vi "Build Send.vi"(4 "BuildType":T2 items=["simple", "Dialog", "PVUpdate", "Dialog&PV", "Asynch", "AsynchDial", "Ack"], 6 "Wiring Spec":T1, 8 "error in (no error)":errorcluster, 10 "Send VI":refnum<vi>, 11 "CS++Actor in":refnum<class "CS++Actor.lvclass">) -> (0 "error out":errorcluster, 3 "CS++Actor out":refnum<class "CS++Actor.lvclass">)   [LabVIEW 2016, in "CS++Actor.lvlib" / "CS++Actor.lvclass"]
doc: "Creates the send.vi of the new message."
uses:
  CS++Actor.lvclass
  CSPP_MessageMakerMain/BuildType.ctl
  <vilib>/LabVIEW Icon API/lv_icon/Controls/Graphic.ctl
  CS++Actor.lvclass/CS++Actor.ctl
  <vilib>/Utility/traverseref.llb/TRef TravTarget.ctl
  <vilib>/Utility/miscctls.llb/LVPositionTypeDef.ctl
  <vilib>/LabVIEW Icon API/lv_icon/Classes/Icon/Icon.lvclass
  <vilib>/LabVIEW Icon API/lv_icon/Classes/Icon Framework/Icon Framework.lvclass
  <vilib>/Utility/traverseref.llb/VI Scripting - Traverse.lvlib
  <vilib>/LabVIEW Icon API/LabVIEW Icon API.lvlib
  CSPP_MessageMakerMain/CS++MessageMakerMain.lvclass
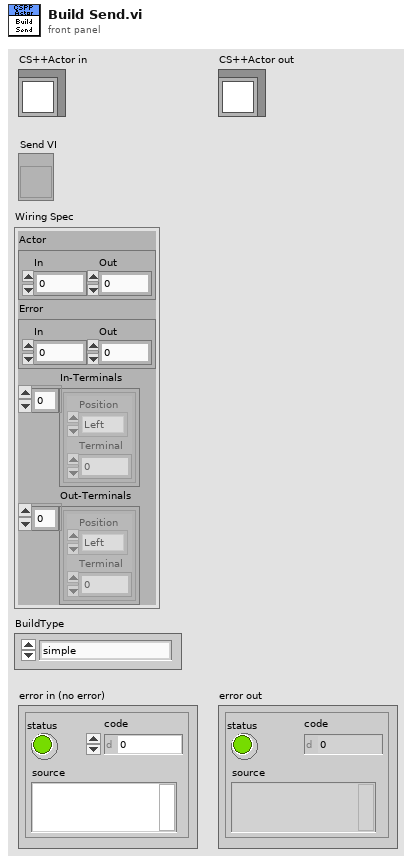
[diagram p1: front panel]
types:
  T1 = cluster{"Actor":cluster{"In":i32, "Out":i32}, "Error":cluster{"In":i32, "Out":i32}, "In-Terminals":cluster{"Position":enum16{"Left", "Top", "Bottom", "Right"}, "Terminal":i32}[], "Out-Terminals":cluster{"Position":enum16{"Left", "Top", "Bottom", "Right"}, "Terminal":i32}[]}
  T2 = typedef "CS++MessageMakerMain.lvlib/CS++MessageMakerMain.lvclass/BuildType.ctl" = u16
  T3 = typedef "Graphic.ctl" = cluster{"Rectangle":cluster{"left":i16, "top":i16, "right":i16, "bottom":i16}, "Path":path, "Image":picture, "Filter":string, "FileName":string}
  T4 = typedef "BodyText.ctl" = cluster{"Line 1 text":string, "Line 2 text":string, "Line 3 text":string, "Line 4 text":string, "Line 1 color":u32, "Line 2 color":u32, "Line 3 color":u32, "Line 4 color":u32, "Body Text Spec":cluster{"Font":T5, "Alignment":T6, "Size":u8}, "Center text vertically":bool, "Capitalize Text":bool}
  T5 = typedef "Font.ctl" = string
  T6 = typedef "Alignment.ctl" = u16
  T7 = typedef "TRef TravTarget.ctl" = enum16{"FP", "BD", "Other"}
  T8 = enum16{"Invalid Wire Rule", "Required", "Recommended", "Optional", "Dynamic Dispatch"}
  T9 = typedef "LVPositionTypeDef.ctl" = cluster{"Left":i32, "Top":i32}
  T10 = enum16{"Invalid Wire Rule", "Required", "Recommended", "Optional", "Dynamic Dispatch"}[]
  T11 = cluster{"Position":enum16{"Left", "Top", "Bottom", "Right"}, "Terminal":i32}[]
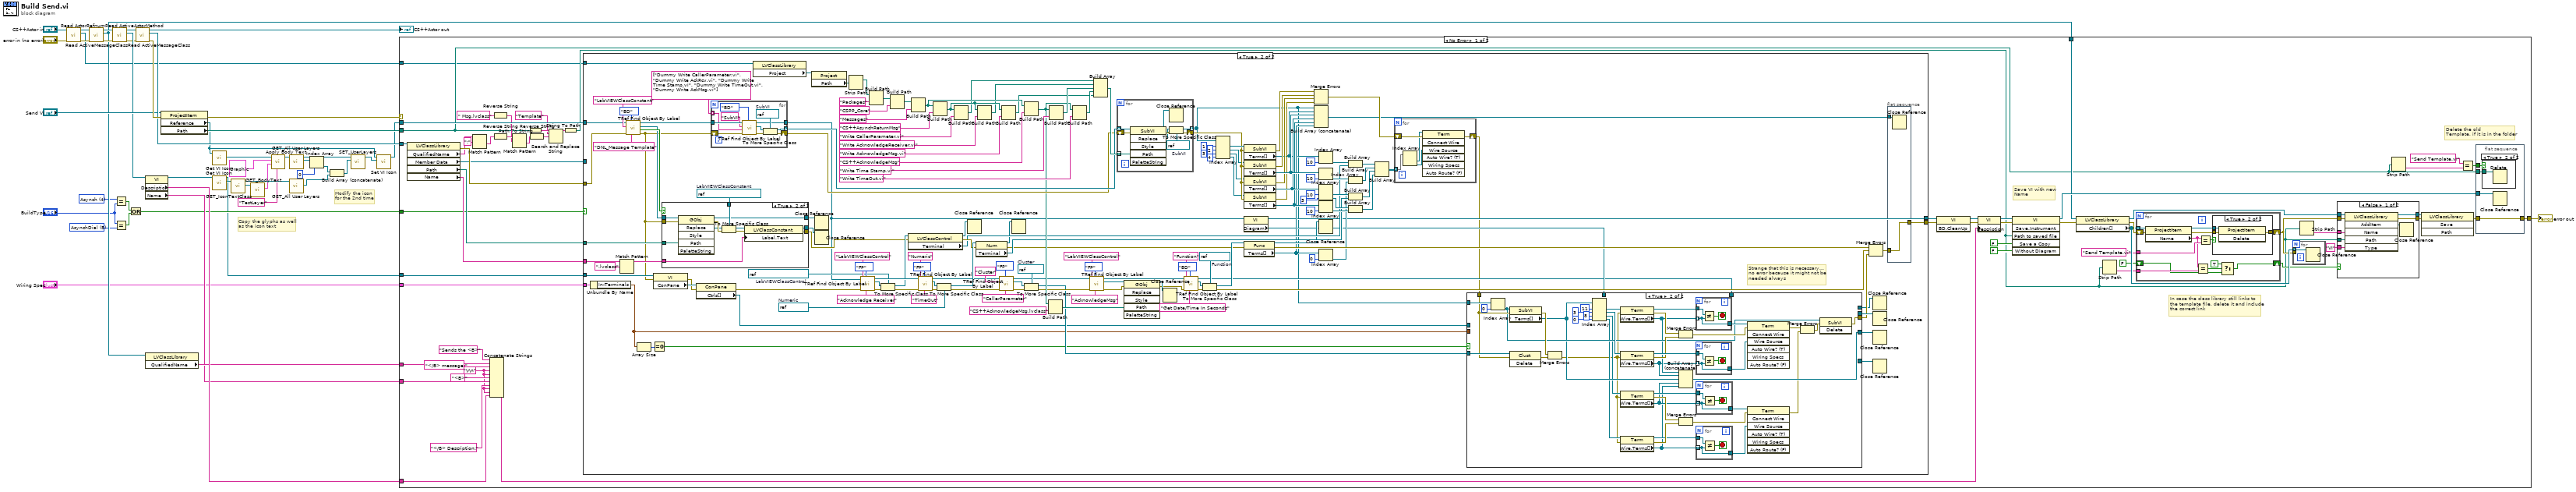
[diagram p0: block diagram]
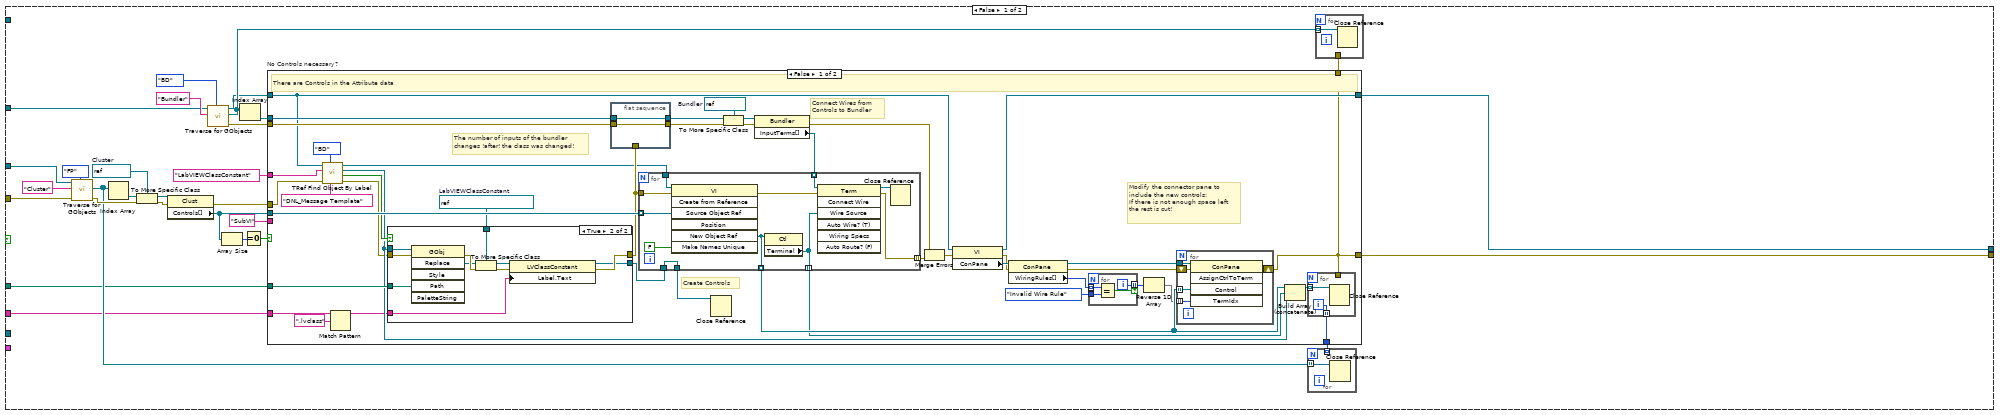
[diagram p3: hidden frame]
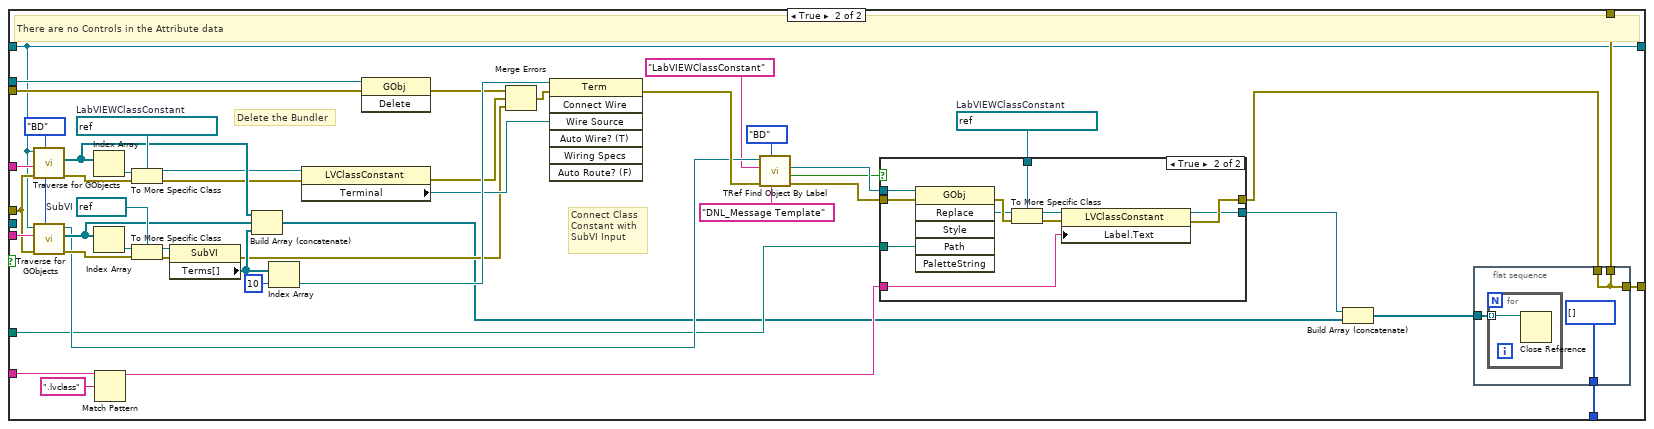
[diagram p5: hidden frame]
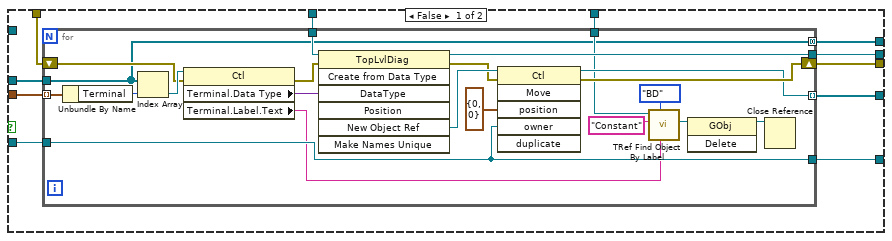
[diagram p8: hidden frame]
diagram:
  w2 = T2 5 items=["simple", "Dialog", "PVUpdate", "Dialog&PV", "Asynch", "AsynchDial", "Ack"] ("BuildType")
  w1 = T2 4 items=["simple", "Dialog", "PVUpdate", "Dialog&PV", "Asynch", "AsynchDial", "Ack"] ("BuildType")
  # "Copy the glyphs as well\nas the icon text"
  # "Modify the icon\nfor the 2nd time"
  n1 = call "Read ActorRefnum.vi"("error in (no error)"="error in (no error)", "CS++Actor in"="CS++Actor in") -> ("error out"=w6:errorcluster, "ActorRefnum"=w5:refnum<vi>, "CS++Actor out"=w8:refnum<class "CS++Actor.lvclass">)  [unwired: 7 in]
  n2 = call "Read ActiveMessageClass.vi"("error in (no error)"=w6, "CS++Actor in"=w8) -> ("error out"=w25:errorcluster, "ActiveMessageClass"=w22:refnum<vi>, "CS++Actor out"=w26:refnum<class "CS++Actor.lvclass">)  [unwired: 7 in]
  n3 = call "Read ActiveActorMethod.vi"("error in (no error)"=w25, "CS++Actor in"=w26) -> ("error out"=w27:errorcluster, "ActiveActorMethod"=w31:refnum<vi>, "CS++Actor out"=w28:refnum<class "CS++Actor.lvclass">)  [unwired: 7 in]
  n4 = Equal?(x=w1, y="BuildType") -> (x = y?=w12:bool)
  n5 = Equal?(x="BuildType", y=w2) -> (x = y?=w11:bool)
  n6 = Or(x=w12, y=w11) -> (x .or. y?=w10:bool)
  n7 = call "Read ActiveMessageClass.vi"("error in (no error)"=w27, "CS++Actor in"=w28) -> ("error out"=w43:errorcluster, "ActiveMessageClass"=w42:refnum<vi>, "CS++Actor out"=→"CS++Actor out":refnum<class "CS++Actor.lvclass">)  [unwired: 7 in]
  n8 = property class="VI"(reference=w31) -> (reference out=w30:refnum<vi>, "Description"=w29:string, "Name"=w23:string)  [unwired: 1 in, 1 out]
  n9 = property class="LVClassLibrary"(reference=w22) -> ("QualifiedName"=w24:string)  [unwired: 1 in, 2 out]
  n10 = property class="ProjectItem"(reference="Send VI", error in=w43) -> (error out=w46:errorcluster, "Reference"=w32:refnum<vi>, "Path"=w45:path)  [unwired: 1 out]
  n11 = call <vilib>:"Get VI Icon.vi"("VI Refnum in"=w32) -> ("Icon"=w18:refnum<class "Icon.lvclass">)  [unwired: 8 in, 2 out]
  n12 = call <vilib>:"Get VI Icon.vi"("VI Refnum in"=w30) -> ("Icon"=w20:refnum<class "Icon.lvclass">, "VI Refnum out"=w3:refnum<vi>)  [unwired: 8 in, 1 out]
  n13 = call-dynamic "GET_IconTextClass.vi"("Icon.lvclass in"=w20) -> ("Icon Framework.lvclass"=w21:refnum<class "Icon Framework.lvclass">, "Icon.lvclass out"=w19:refnum<class "Icon.lvclass">)  [unwired: 8 in, 1 out]
  n14 = call-dynamic "GET_BodyText.vi"("Icon Framework.lvclass in"=w21) -> ("Body Text"=w16:T4)  [unwired: 7 in, 3 out]
  n15 = call <vilib>:"Apply Body Text.vi"("Layer name"="TestLayer", "Body test"=w16, "Path & Icon"=T3 {"Rectangle"={"left"=0, "top"=0, "right"=0, "bottom"=0}, "Path"=path "", "Image"=bytes[0], "Filter"="", "FileName"=""}, "Icon in"=w18) -> ("Icon out"=w17:refnum<class "Icon.lvclass">)  [unwired: 5 in, 2 out]
  n16 = call-dynamic "GET_All User Layers.vi"("Icon.lvclass in"=w17) -> ("User Layer"=w39:refnum<class "Layer.lvclass">[], "Icon.lvclass out"=w40:refnum<class "Icon.lvclass">)  [unwired: 8 in, 1 out]
  n17 = call-dynamic "GET_All User Layers.vi"("Icon.lvclass in"=w19) -> ("User Layer"=w36:refnum<class "Layer.lvclass">[])  [unwired: 8 in, 2 out]
  n18 = Index Array(array=w39, index=0) -> (element=w37:refnum<class "Layer.lvclass">)
  n19 = Build Array (concatenate)(w37, w36) -> (w35:refnum<class "Layer.lvclass">[])
  n20 = call-dynamic "SET_UserLayers.vi"("Layers"=w35, "Icon.lvclass in"=w40) -> ("Icon.lvclass out"=w34:refnum<class "Icon.lvclass">)  [unwired: 8 in, 1 out]
  n21 = call <vilib>:"Set VI Icon.vi"("Icon"=w34, "VI Refnum in"=w32) -> ("VI Refnum out"=w33:refnum<vi>)  [unwired: 8 in, 1 out]
  n22 = case shown="No Error" w46 {
    selector: w46 -> [_ w596]
    tunnel: [w59 w596] -> w47
    tunnel: w42 -> [w60 _]
    tunnel: w33 -> [w106 _]
    tunnel: w45 -> [w57 _]
    tunnel: w29 -> [w80 _]
    tunnel: w24 -> [w72 _]
    tunnel: w23 -> [w83 _]
    tunnel: w22 -> [w75 _]
    tunnel: w10 -> [w51 _]
    tunnel: w5 -> [w50 _]
    tunnel: "Wiring Spec" -> [w49 _]
    tunnel: w3 -> [w48 _]
    frame No Error {
      w79 = "\r\n"
      # "In case the class library still links to\nthe template file, delete it and include\nthe correct link"
      # "Delete the old\nTemplate, if it is in the folder"
      # "Save VI with new\nName"
      n23 = property class="LVClassLibrary"(reference=w60) -> (error out=w107:errorcluster, "QualifiedName"=w100:string, "Member Data"=w101:refnum<vi>, "Path"=w62:path, "Name"=w52:string)  [unwired: 1 in, 1 out]
      n24 = Match Pattern(string=w100, regular expression=":") -> (after substring=w93:string)  [unwired: 1 in, 3 out]
      n25 = Concatenate Strings("Sends the <B>", w72, "</B> message.", w79, w79, "<B>" ("string"), w83, "</B> Description:" ("string"), w79, w79, w80) -> (w86:string)
      n26 = Reverse String(1:" Msg.lvclass" ("search string")) -> (0:w95:string)
      n27 = Reverse String(1:w93) -> (0:w97:string)
      n28 = Match Pattern(string=w97, regular expression=w95) -> (after substring=w96:string)  [unwired: 1 in, 3 out]
      n29 = Path To String(path=w57) -> (string=w104:string)
      n30 = Reverse String(1:w96) -> (0:w98:string)
      n31 = Search and Replace String(input string=w104, search string="Template", replace string=w98) -> (result string=w102:string)  [unwired: 5 in, 3 out]
      n32 = String To Path(string=w102) -> (path=w61:path)
      n33 = case shown="True" w51 {
        tunnel: w107 -> [w136 w438]
        tunnel: w106 -> [w125 w440]
        tunnel: w101 -> [w124 _]
        tunnel: [w123 w288] -> w91
        tunnel: w62 -> [w116 w432]
        tunnel: [w114 w304] -> w53
        tunnel: w52 -> [w113 w434]
        tunnel: w50 -> [_ w428]
        tunnel: w49 -> [_ w321]
        tunnel: w48 -> [_ w320]
        frame False {
          w138 = refnum<vi> refnum  # Cluster
          n34 = call <vilib>:"Traverse for GObjects.vi"("Traverse Target"=TRef_TravTarget."FP", "error in (no error)"=w136, "Class Name"="Cluster" ("name/order"), "VI Refnum"=w124) -> ("error out"=w137:errorcluster, "References"=w128:refnum<vi>[])  [unwired: 4 in, 2 out]
          n35 = Index Array(array=w128) -> (element=w139:refnum<vi>)  [unwired: 1 in]
          n36 = To More Specific Class(target class=w138, reference=w139, error in=w137) -> (specific class reference=w135:refnum<vi>, error out=w134:errorcluster)
          n37 = property class="Clust"(reference=w135, error in=w134) -> (error out=w133:errorcluster, "Controls[]"=w122:refnum<vi>[])  [unwired: 1 out]
          n38 = call <vilib>:"Traverse for GObjects.vi"("Traverse Target"=TRef_TravTarget."BD", "Class Name"="Bundler", "VI Refnum"=w125) -> ("error out"=w130:errorcluster, "References"=w127:refnum<vi>[], "dup VI Refnum"=w115:refnum<vi>)  [unwired: 5 in, 1 out]
          n39 = Array Size(array=w122) -> (size(s)=w121:i32)
          n40 = Index Array(array=w127) -> (element=w120:refnum<vi>)  [unwired: 1 in]
          n41 = Equal To 0?(x=w121) -> (x = 0?=w119:bool)
          n42 = case "No Controls necessary?" shown="False" w119 {
            tunnel: w133 -> [w159 w256]
            tunnel: w130 -> [w145 w266]
            tunnel: [w179 w263] -> w129
            tunnel: [w163 w264] -> w126
            tunnel: [w163 w265] -> w123
            tunnel: w122 -> [w164 _]
            tunnel: w120 -> [w147 w267]
            tunnel: "LabVIEWClassConstant" ("Class Name") -> [w155 w262]
            tunnel: "SubVI" ("Class Name") -> [_ w257]
            tunnel: w116 -> [w176 w225]
            tunnel: w115 -> [w142 w221]
            tunnel: [w169 w221] -> w114
            tunnel: w113 -> [w151 w227]
            frame False {
              w149 = refnum<vi> refnum  # LabVIEWClassConstant
              w184 = refnum<vi> refnum  # Bundler
              # "The number of inputs of the bundler\nchanges !after! the class was changed!"
              # "Modify the connector pane to\ninclude the new controls:\nIf there is not enough space left\nthe rest is cut!"
              # "Connect Wires from\nControls to Bundler"
              # "Create Controls"
              # "There are Controls in the Attribute data"
              n43 = call <vilib>:"TRef Find Object By Label.vi"("Label"="DNL_Message Template", "Traverse Target"=TRef_TravTarget."BD", "error in (no error)"=w159, "Class Name"=w155, "VI Ref"=w142) -> ("error out"=w153:errorcluster, "Found?"=w156:bool, "Found Obj Ref"=w154:refnum<vi>, "dup VI Ref"=w143:refnum<vi>)  [unwired: 3 in]
              n44 = Match Pattern(string=w151, regular expression=".lvclass") -> (before substring=w150:string)  [unwired: 1 in, 3 out]
              n45 = case shown="True" w156 {
                tunnel: [w187 w192] -> w144
                tunnel: w176 -> [_ w198]
                tunnel: [_ w190] -> w175
                tunnel: w154 -> [_ w196]
                tunnel: w153 -> [w187 w197]
                tunnel: w150 -> [_ w188]
                tunnel: w149 -> [_ w189]
                frame False {
                }
                frame True {
                  n46 = invoke class="GObj" method="Replace"(reference=w196, error in=w197, "Path"=w198) -> (error out=w195:errorcluster, "Replace"=w194:refnum<vi>)  [unwired: 3 in, 4 out]
                  n47 = To More Specific Class(target class=w189, reference=w194, error in=w195) -> (specific class reference=w191:refnum<vi>, error out=w193:errorcluster)
                  n48 = property class="LVClassConstant"(reference=w191, error in=w193, "Label.Text"=w188) -> (reference out=w190:refnum<vi>, error out=w192:errorcluster)
                }
              }
              n49 = flat-sequence {
                tunnel: [w186] -> w148
                tunnel: w147 -> [w186]
                tunnel: [w185] -> w146
                tunnel: w145 -> [w185]
                tunnel: w144 -> [_]
                frame #0 {
                }
              }
              n50 = To More Specific Class(target class=w184, reference=w148, error in=w146) -> (specific class reference=w183:refnum<vi>, error out=w182:errorcluster)
              n51 = property class="Bundler"(reference=w183, error in=w182) -> (error out=w178:errorcluster, "InputTerms[]"=w181:refnum<vi>[])  [unwired: 1 out]
              n52 = for {
                tunnel: w164 -> [w220] mode=indexing
                tunnel: w143 -> [w218]
                tunnel: w144 -> [w217]
                tunnel: w181 -> [w215] mode=indexing
                tunnel: [w214] -> w180 mode=indexing
                tunnel: [w213] -> w161 mode=indexing
                tunnel: w175 -> [w211]
                tunnel: [w211] -> w174
                tunnel: [w210] -> w162 mode=indexing
                n53 = invoke class="VI" method="Create from Reference"(reference=w218, error in=w217, "Source Object Ref"=w220, "Make Names Unique"=FALSE ("Make Names Unique (F)")) -> (error out=w216:errorcluster, "New Object Ref"=w210:refnum<vi>)  [unwired: 3 in, 5 out]
                n54 = property class="Ctl"(reference=w210) -> ("Terminal"=w213:refnum<vi>)  [unwired: 1 in, 2 out]
                n55 = invoke class="Term" method="Connect Wire"(reference=w215, error in=w216, "Wire Source"=w213) -> (reference out=w212:refnum<vi>, error out=w214:errorcluster)  [unwired: 4 in, 5 out]
                n56 = Close Reference(reference=w212) -> ()  [unwired: 1 in, 1 out]
              }
              n57 = Close Reference(reference=w174) -> ()  [unwired: 1 in, 1 out]
              n58 = Merge Errors(w178, w180) -> (w173:errorcluster)
              n59 = property class="VI"(reference=w142, error in=w173) -> (reference out=w169:refnum<vi>, error out=w170:errorcluster, "ConPane"=w172:refnum<vi>)
              n60 = property class="ConPane"(reference=w172, error in=w170) -> (reference out=w171:refnum<vi>, error out=w166:errorcluster, "WiringRules[]"=w168:T10)
              n61 = for {
                tunnel: w168 -> [w207] mode=indexing
                tunnel: T8."Invalid Wire Rule" ("Wire Rule") -> [w206]
                tunnel: [w205] -> w165 mode=indexing if=w204
                i -> [w205]
                n62 = Equal?(x=w207, y=w206) -> (x = y?=w204:bool)
              }
              n63 = Reverse 1D Array(array=w165) -> (reversed array=w160:i32[])
              n64 = for {
                tunnel: w171 -> [w203]
                shift-right: [w201] -> w163
                shift-left: w166 -> [w202]
                tunnel: w160 -> [w200] mode=indexing
                tunnel: w162 -> [w199] mode=indexing
                n65 = invoke class="ConPane" method="AssignCtrlToTerm"(reference=w203, error in=w202, "Control"=w199, "TermIdx"=w200) -> (error out=w201:errorcluster)  [unwired: 1 in, 4 out]
              }
              n66 = Build Array (concatenate)(w162, w161, w154) -> (w177:refnum<vi>[])
              n67 = for {
                tunnel: w177 -> [w209] mode=indexing
                tunnel: [w208] -> w179 mode=indexing
                tunnel: w163 -> [_]
                i -> [w208]
                n68 = Close Reference(reference=w209) -> ()  [unwired: 1 in, 1 out]
              }
            }
            frame True {
              w234 = refnum<vi> refnum  # LabVIEWClassConstant
              w253 = refnum<vi> refnum  # SubVI
              w260 = refnum<vi> refnum  # LabVIEWClassConstant
              w258 = TRef_TravTarget."BD" ("Traverse Target")
              # "Connect Class\nConstant with\nSubVI Input"
              # "Delete the Bundler"
              # "There are no Controls in the Attribute data"
              n69 = call <vilib>:"Traverse for GObjects.vi"("Traverse Target"=w258, "error in (no error)"=w256, "Class Name"=w262, "VI Refnum"=w221) -> ("error out"=w259:errorcluster, "References"=w246:refnum<vi>[])  [unwired: 4 in, 2 out]
              n70 = call <vilib>:"Traverse for GObjects.vi"("Traverse Target"=w258, "error in (no error)"=w256, "Class Name"=w257, "VI Refnum"=w221) -> ("error out"=w254:errorcluster, "References"=w245:refnum<vi>[], "dup VI Refnum"=w230:refnum<vi>)  [unwired: 4 in, 1 out]
              n71 = Index Array(array=w246) -> (element=w261:refnum<vi>)  [unwired: 1 in]
              n72 = Index Array(array=w245) -> (element=w255:refnum<vi>)  [unwired: 1 in]
              n73 = Match Pattern(string=w227, regular expression=".lvclass") -> (before substring=w226:string)  [unwired: 1 in, 3 out]
              n74 = To More Specific Class(target class=w260, reference=w261, error in=w259) -> (specific class reference=w243:refnum<vi>, error out=w241:errorcluster)
              n75 = To More Specific Class(target class=w253, reference=w255, error in=w254) -> (specific class reference=w252:refnum<vi>, error out=w251:errorcluster)
              n76 = property class="SubVI"(reference=w252, error in=w251) -> (error out=w239:errorcluster, "Terms[]"=w244:refnum<vi>[])  [unwired: 1 out]
              n77 = Build Array (concatenate)(w246, w245, w244) -> (w223:refnum<vi>[])
              n78 = Index Array(array=w244, index=10) -> (element=w249:refnum<vi>)
              n79 = property class="LVClassConstant"(reference=w243, error in=w241) -> (error out=w240:errorcluster, "Terminal"=w242:refnum<vi>)  [unwired: 1 out]
              n80 = invoke class="GObj" method="Delete"(reference=w267, error in=w266) -> (error out=w248:errorcluster)  [unwired: 1 in, 2 out]
              n81 = Merge Errors(w248, w240, w239) -> (w247:errorcluster)
              n82 = invoke class="Term" method="Connect Wire"(reference=w249, error in=w247, "Wire Source"=w242) -> (error out=w232:errorcluster)  [unwired: 4 in, 6 out]
              n83 = call <vilib>:"TRef Find Object By Label.vi"("Label"="DNL_Message Template", "Traverse Target"=TRef_TravTarget."BD", "error in (no error)"=w232, "Class Name"="LabVIEWClassConstant", "VI Ref"=w230) -> ("error out"=w233:errorcluster, "Found?"=w237:bool, "Found Obj Ref"=w238:refnum<vi>)  [unwired: 3 in, 1 out]
              n84 = case shown="True" w237 {
                tunnel: [w268 w273] -> w231
                tunnel: w225 -> [_ w279]
                tunnel: [_ w271] -> w224
                tunnel: w238 -> [_ w277]
                tunnel: w233 -> [w268 w278]
                tunnel: w226 -> [_ w269]
                tunnel: w234 -> [_ w270]
                frame False {
                }
                frame True {
                  n85 = invoke class="GObj" method="Replace"(reference=w277, error in=w278, "Path"=w279) -> (error out=w276:errorcluster, "Replace"=w275:refnum<vi>)  [unwired: 3 in, 4 out]
                  n86 = To More Specific Class(target class=w270, reference=w275, error in=w276) -> (specific class reference=w272:refnum<vi>, error out=w274:errorcluster)
                  n87 = property class="LVClassConstant"(reference=w272, error in=w274, "Label.Text"=w269) -> (reference out=w271:refnum<vi>, error out=w273:errorcluster)
                }
              }
              n88 = Build Array (concatenate)(w224, w223) -> (w222:refnum<vi>[])
              n89 = flat-sequence {
                tunnel: [w280] -> w265
                tunnel: [w280] -> w264
                tunnel: [i32[] []] -> w263
                tunnel: w231 -> [w280]
                tunnel: w222 -> [w281]
                frame #0 {
                  n90 = for {
                    tunnel: w281 -> [w283] mode=indexing
                    n91 = Close Reference(reference=w283) -> ()  [unwired: 1 in, 1 out]
                  }
                }
              }
            }
          }
          n92 = for {
            tunnel: w128 -> [w285] mode=indexing
            tunnel: w129 -> [_] mode=indexing
            n93 = Close Reference(reference=w285) -> ()  [unwired: 1 in, 1 out]
          }
          n94 = for {
            tunnel: w127 -> [w284] mode=indexing
            tunnel: w126 -> [_]
            n95 = Close Reference(reference=w284) -> ()  [unwired: 1 in, 1 out]
          }
        }
        frame True {
          w314 = refnum<vi> refnum  # Cluster
          w337 = refnum<vi> refnum  # Function
          w350 = refnum<vi> refnum  # Numeric
          w351 = refnum<vi> refnum  # LabVIEWClassControl
          w435 = refnum<vi> refnum  # LabVIEWClassConstant
          # "Strange that this is necessary...\nno error because it might not be\nneeded always"
          n96 = Unbundle By Name(w321) -> ("In-Terminals"=w294:T11)
          n97 = Match Pattern(string=w434, regular expression=".lvclass") -> (before substring=w436:string)  [unwired: 1 in, 3 out]
          n98 = call <vilib>:"TRef Find Object By Label.vi"("Label"="DNL_Message Template", "Traverse Target"=TRef_TravTarget."BD", "error in (no error)"=w438, "Class Name"="LabVIEWClassConstant", "VI Ref"=w440) -> ("error out"=w317:errorcluster, "Found?"=w433:bool, "Found Obj Ref"=w431:refnum<vi>, "dup VI Ref"=w429:refnum<vi>)  [unwired: 3 in]
          n99 = Array Size(array=w294) -> (size(s)=w293:i32)
          n100 = Equal To 0?(x=w293) -> (x = 0?=w291:bool)
          n101 = property class="VI"(reference=w320, error in=w317) -> (error out=w318:errorcluster, "ConPane"=w319:refnum<vi>)  [unwired: 1 out]
          n102 = case shown="True" w433 {
            tunnel: [w471 w477] -> w349
            tunnel: w432 -> [_ w483]
            tunnel: [_ w475] -> w401
            tunnel: w431 -> [w470 w481]
            tunnel: w317 -> [w471 w482]
            tunnel: w436 -> [_ w473]
            tunnel: w435 -> [_ w474]
            tunnel: [w470 w472] -> w402
            frame False {
            }
            frame True {
              n103 = invoke class="GObj" method="Replace"(reference=w481, error in=w482, "Path"=w483) -> (reference out=w472:refnum<vi>, error out=w480:errorcluster, "Replace"=w479:refnum<vi>)  [unwired: 3 in, 3 out]
              n104 = To More Specific Class(target class=w474, reference=w479, error in=w480) -> (specific class reference=w476:refnum<vi>, error out=w478:errorcluster)
              n105 = property class="LVClassConstant"(reference=w476, error in=w478, "Label.Text"=w473) -> (reference out=w475:refnum<vi>, error out=w477:errorcluster)
            }
          }
          n106 = property class="ConPane"(reference=w319, error in=w318) -> (error out=w316:errorcluster, "Ctrls[]"=w297:refnum<vi>[])  [unwired: 1 out]
          n107 = for {
            tunnel: w429 -> [w469]
            tunnel: string[] ["Dummy Write CallerParameter.vi", "Dummy Write AckRcv.vi", "Dummy Write Time Stamp.vi", "Dummy Write TimeOut.vi", "Dummy Write AckMsg.vi"] -> [w465] mode=indexing
            shift-right: [w462] -> w403
            shift-left: w317 -> [w466]
            tunnel: [w460] -> w404 mode=indexing
            tunnel: [w459] -> w303
            w461 = refnum<vi> refnum  # SubVI
            n108 = call <vilib>:"TRef Find Object By Label.vi"("Label"=w465, "Traverse Target"=TRef_TravTarget."BD", "error in (no error)"=w466, "Class Name"="SubVI", "VI Ref"=w469) -> ("error out"=w464:errorcluster, "Found Obj Ref"=w463:refnum<vi>, "dup VI Ref"=w459:refnum<vi>)  [unwired: 3 in, 1 out]
            n109 = To More Specific Class(target class=w461, reference=w463, error in=w464) -> (specific class reference=w460:refnum<vi>, error out=w462:errorcluster)
          }
          n110 = property class="LVClassLibrary"(reference=w428) -> ("Project"=w427:refnum<vi>)  [unwired: 1 in, 2 out]
          n111 = property class="Project"(reference=w427) -> ("Path"=w416:path)  [unwired: 1 in, 2 out]
          n112 = Close Reference(reference=w402) -> ()  [unwired: 1 in, 1 out]
          n113 = Close Reference(reference=w401) -> ()  [unwired: 1 in, 1 out]
          n114 = Strip Path(path=w416) -> (stripped path=w415:path)  [unwired: 1 out]
          n115 = call <vilib>:"TRef Find Object By Label.vi"("Label"="Acknowledge Receiver", "Traverse Target"=TRef_TravTarget."FP", "error in (no error)"=w316, "Class Name"="LabVIEWClassControl", "VI Ref"=w303) -> ("error out"=w356:errorcluster, "Found Obj Ref"=w354:refnum<vi>, "dup VI Ref"=w384:refnum<vi>)  [unwired: 3 in, 1 out]
          n116 = Build Path(base path=w415, name or relative path="Packages") -> (appended path=w425:path)
          n117 = To More Specific Class(target class=w351, reference=w354, error in=w356) -> (specific class reference=w353:refnum<vi>, error out=w355:errorcluster)
          n118 = Build Path(base path=w425, name or relative path="CSPP_Core") -> (appended path=w417:path)
          n119 = property class="LVClassControl"(reference=w353, error in=w349) -> (reference out=w346:refnum<vi>, error out=w352:errorcluster, "Terminal"=w347:refnum<vi>)
          n120 = Build Path(base path=w417, name or relative path="Messages") -> (appended path=w414:path)
          n121 = call <vilib>:"TRef Find Object By Label.vi"("Label"="TimeOut", "Traverse Target"=TRef_TravTarget."FP", "error in (no error)"=w355, "Class Name"="Numeric", "VI Ref"=w384) -> ("error out"=w359:errorcluster, "Found Obj Ref"=w358:refnum<vi>, "dup VI Ref"=w308:refnum<vi>)  [unwired: 3 in, 1 out]
          n122 = Build Path(base path=w414, name or relative path="CS++AsynchReturnMsg") -> (appended path=w418:path)
          n123 = To More Specific Class(target class=w350, reference=w358, error in=w359) -> (specific class reference=w357:refnum<vi>, error out=w307:errorcluster)
          n124 = Build Path(base path=w418, name or relative path="Write CallerParameter.vi") -> (appended path=w410:path)
          n125 = Close Reference(reference=w346) -> ()  [unwired: 1 in, 1 out]
          n126 = property class="Num"(reference=w357, error in=w352) -> (reference out=w345:refnum<vi>, error out=w335:errorcluster, "Terminal"=w348:refnum<vi>)
          n127 = Build Path(base path=w418, name or relative path="Write AcknowledgeReceiver.vi") -> (appended path=w409:path)
          n128 = call <vilib>:"TRef Find Object By Label.vi"("Label"="CallerParameter", "Traverse Target"=TRef_TravTarget."FP", "error in (no error)"=w307, "Class Name"="Cluster", "VI Ref"=w308) -> ("error out"=w312:errorcluster, "Found Obj Ref"=w313:refnum<vi>, "dup VI Ref"=w305:refnum<vi>)  [unwired: 3 in, 1 out]
          n129 = Build Path(base path=w418, name or relative path="Write AcknowledgeMsg.vi") -> (appended path=w406:path)
          n130 = Close Reference(reference=w345) -> ()  [unwired: 1 in, 1 out]
          n131 = To More Specific Class(target class=w314, reference=w313, error in=w312) -> (specific class reference=w300:refnum<vi>, error out=w306:errorcluster)
          n132 = Build Path(base path=w414, name or relative path="CS++AcknowledgeMsg") -> (appended path=w393:path)
          n133 = Build Path(base path=w393, name or relative path="CS++AcknowledgeMsg.lvclass") -> (appended path=w394:path)
          n134 = Build Path(base path=w393, name or relative path="Write Time Stamp.vi") -> (appended path=w408:path)
          n135 = Build Path(base path=w393, name or relative path="Write TimeOut.vi") -> (appended path=w407:path)
          n136 = call <vilib>:"TRef Find Object By Label.vi"("Label"="AcknowledgeMsg", "Traverse Target"=TRef_TravTarget."FP", "error in (no error)"=w306, "Class Name"="LabVIEWClassControl", "VI Ref"=w305) -> ("error out"=w396:errorcluster, "Found Obj Ref"=w397:refnum<vi>, "dup VI Ref"=w338:refnum<vi>)  [unwired: 3 in, 1 out]
          n137 = Build Array(w410, w409, w408, w407, w406) -> (w405:path[])
          n138 = for {
            shift-right: [w454] -> w377
            shift-left: w403 -> [w458]
            tunnel: w404 -> [w457] mode=indexing
            tunnel: w405 -> [w456] mode=indexing
            tunnel: [w452] -> w286 mode=indexing
            w451 = refnum<vi> refnum  # SubVI
            n139 = invoke class="SubVI" method="Replace"(reference=w457, error in=w458, "Path"=w456) -> (reference out=w450:refnum<vi>, error out=w455:errorcluster, "Replace"=w453:refnum<vi>)  [unwired: 3 in, 3 out]
            n140 = Close Reference(reference=w450) -> ()  [unwired: 1 in, 1 out]
            n141 = To More Specific Class(target class=w451, reference=w453, error in=w455) -> (specific class reference=w452:refnum<vi>, error out=w454:errorcluster)
          }
          n142 = invoke class="GObj" method="Replace"(reference=w397, error in=w396, "Path"=w394) -> (reference out=w392:refnum<vi>, error out=w339:errorcluster)  [unwired: 3 in, 4 out]
          n143 = Close Reference(reference=w392) -> ()  [unwired: 1 in, 1 out]
          n144 = call <vilib>:"TRef Find Object By Label.vi"("Label"="Get Date/Time In Seconds", "Traverse Target"=TRef_TravTarget."BD", "error in (no error)"=w339, "Class Name"="Function", "VI Ref"=w338) -> ("error out"=w343:errorcluster, "Found Obj Ref"=w344:refnum<vi>, "dup VI Ref"=w295:refnum<vi>)  [unwired: 3 in, 1 out]
          n145 = To More Specific Class(target class=w337, reference=w344, error in=w343) -> (specific class reference=w336:refnum<vi>, error out=w315:errorcluster)
          n146 = Index Array(array=w286, index #1=1 ("index"), index #2=2 ("index"), index #3=3 ("index"), index #4=4 ("index")) -> (element #1=w378:refnum<vi>, element #2=w376:refnum<vi>, element #3=w375:refnum<vi>, element #4=w374:refnum<vi>)
          n147 = property class="SubVI"(reference=w378, error in=w377) -> (error out=w326:errorcluster, "Terms[]"=w287:refnum<vi>[])  [unwired: 1 out]
          n148 = property class="SubVI"(reference=w376, error in=w377) -> (error out=w325:errorcluster, "Terms[]"=w330:refnum<vi>[])  [unwired: 1 out]
          n149 = property class="SubVI"(reference=w375, error in=w377) -> (error out=w324:errorcluster, "Terms[]"=w329:refnum<vi>[])  [unwired: 1 out]
          n150 = property class="SubVI"(reference=w374, error in=w377) -> (error out=w323:errorcluster, "Terms[]"=w328:refnum<vi>[])  [unwired: 1 out]
          n151 = property class="VI"(reference=w303) -> (reference out=w304:refnum<vi>, "Diagram"=w302:refnum<vi>)  [unwired: 1 in, 1 out]
          n152 = property class="Func"(reference=w336, error in=w335) -> (reference out=w333:refnum<vi>, error out=w334:errorcluster, "Terms[]"=w327:refnum<vi>[])
          n153 = Merge Errors(w326, w325, w324, w323) -> (w369:errorcluster)
          n154 = Build Array (concatenate)(w286, w287, w330, w329, w328, w327) -> (w322:refnum<vi>[])
          n155 = Index Array(array=w287, index=10) -> (element=w361:refnum<vi>)
          n156 = Index Array(array=w330, index=10) -> (element=w367:refnum<vi>)
          n157 = Index Array(array=w329, index #1=10 ("index"), index #2=3 ("index")) -> (element #1=w360:refnum<vi>, element #2=w364:refnum<vi>)
          n158 = Index Array(array=w328, index=10) -> (element=w365:refnum<vi>)
          n159 = Close Reference(reference=w333) -> ()  [unwired: 1 in, 1 out]
          n160 = Index Array(array=w327, index=0) -> (element=w331:refnum<vi>)
          n161 = Build Array(w361, w347) -> (w368:refnum<vi>[])
          n162 = Build Array(w367, w331) -> (w366:refnum<vi>[])
          n163 = Build Array(w360, w348) -> (w363:refnum<vi>[])
          n164 = Build Array(w364, w365) -> (w362:refnum<vi>[])
          n165 = Build Array(w368, w366, w363, w362) -> (w388:refnum<vi>[][])
          n166 = for {
            shift-right: [w448] -> w290
            shift-left: w369 -> [w449]
            tunnel: w388 -> [w447] mode=indexing
            n167 = Index Array(array=w447) -> (element #1=w446:refnum<vi>, element #2=w445:refnum<vi>)  [unwired: 2 in]
            n168 = invoke class="Term" method="Connect Wire"(reference=w446, error in=w449, "Wire Source"=w445) -> (error out=w448:errorcluster)  [unwired: 4 in, 6 out]
          }
          n169 = case shown="True" w291 {
            tunnel: w302 -> [w494 _]
            tunnel: [w493 _] -> w301
            tunnel: w300 -> [w492 w555]
            tunnel: [w491 _] -> w299
            tunnel: [w490 w538] -> w298
            tunnel: w297 -> [w489 _]
            tunnel: [w488 w533] -> w296
            tunnel: w295 -> [w487 _]
            tunnel: w294 -> [w486 _]
            tunnel: w290 -> [w485 w546]
            tunnel: [w484 _] -> w292
            tunnel: w286 -> [_ w547]
            frame False {
              n170 = for {
                tunnel: w489 -> [w495]
                tunnel: w486 -> [w513] mode=indexing
                shift-right: [w504] -> w490
                shift-left: w485 -> [w510]
                tunnel: w494 -> [w509]
                tunnel: [w508] -> w493
                tunnel: w492 -> [w503]
                tunnel: [w503] -> w491
                tunnel: [w502] -> w488 mode=indexing
                tunnel: w487 -> [w498]
                tunnel: [w495] -> w484 mode=concatenating
                n171 = Unbundle By Name(w513) -> ("Terminal"=w512:i32)
                n172 = Index Array(array=w495, index=w512) -> (element=w511:refnum<vi>)
                n173 = property class="Ctl"(reference=w511, error in=w510) -> (error out=w514:errorcluster, "Terminal.Data Type"=w515:variant, "Terminal.Label.Text"=w499:string)  [unwired: 1 out]
                n174 = invoke class="TopLvlDiag" method="Create from Data Type"(reference=w509, error in=w514, "DataType"=w515) -> (reference out=w508:refnum<vi>, error out=w505:errorcluster, "New Object Ref"=w506:refnum<vi>)  [unwired: 4 in, 4 out]
                n175 = invoke class="Ctl" method="Move"(reference=w506, error in=w505, "position"=T9 {"Left"=0, "Top"=0}, "owner"=w503) -> (reference out=w502:refnum<vi>, error out=w504:errorcluster)  [unwired: 2 in, 4 out]
                n176 = call <vilib>:"TRef Find Object By Label.vi"("Label"=w499, "Traverse Target"=TRef_TravTarget."BD", "Class Name"="Constant", "VI Ref"=w498) -> ("Found Obj Ref"=w497:refnum<vi>)  [unwired: 4 in, 3 out]
                n177 = invoke class="GObj" method="Delete"(reference=w497) -> (reference out=w496:refnum<vi>)  [unwired: 2 in, 2 out]
                n178 = Close Reference(reference=w496) -> ()  [unwired: 1 in, 1 out]
              }
            }
            frame True {
              n179 = Index Array(array=w547, index=0) -> (element=w537:refnum<vi>)
              n180 = property class="SubVI"(reference=w537, error in=w546) -> (error out=w545:errorcluster, "Terms[]"=w534:refnum<vi>[])  [unwired: 1 out]
              n181 = invoke class="Clust" method="Delete"(reference=w555, error in=w546) -> (error out=w544:errorcluster)  [unwired: 1 in, 2 out]
              n182 = Merge Errors(w545, w544) -> (w526:errorcluster)
              n183 = Index Array(array=w534, index #1=11 ("index"), index #2=3 ("index"), index #3=8 ("index"), index #4=0 ("index")) -> (element #1=w551:refnum<vi>, element #2=w552:refnum<vi>, element #3=w528:refnum<vi>, element #4=w527:refnum<vi>)
              n184 = property class="Term"(reference=w551, error in=w526) -> (reference out=w549:refnum<vi>, error out=w541:errorcluster, "Wire.Terms[]"=w536:refnum<vi>[])
              n185 = property class="Term"(reference=w552, error in=w526) -> (reference out=w550:refnum<vi>, error out=w540:errorcluster, "Wire.Terms[]"=w535:refnum<vi>[])
              n186 = property class="Term"(reference=w528, error in=w526) -> (reference out=w518:refnum<vi>, error out=w525:errorcluster, "Wire.Terms[]"=w517:refnum<vi>[])
              n187 = property class="Term"(reference=w527, error in=w526) -> (reference out=w519:refnum<vi>, error out=w524:errorcluster, "Wire.Terms[]"=w516:refnum<vi>[])
              n188 = Merge Errors(w541, w540) -> (w539:errorcluster)
              n189 = Build Array (concatenate)(w536, w535, w534, w517, w516) -> (w533:refnum<vi>[])
              n190 = Merge Errors(w525, w524) -> (w523:errorcluster)
              n191 = for {
                tunnel: w536 -> [w562] mode=indexing
                tunnel: w549 -> [w564]
                tunnel: [w562] -> w543
                stop <- w563 stop-if-true
                n192 = Not Equal?(x=w564, y=w562) -> (x != y?=w563:bool)
              }
              n193 = for {
                tunnel: w535 -> [w565] mode=indexing
                tunnel: w550 -> [w567]
                tunnel: [w565] -> w542
                stop <- w566 stop-if-true
                n194 = Not Equal?(x=w567, y=w565) -> (x != y?=w566:bool)
              }
              n195 = for {
                tunnel: w517 -> [w556] mode=indexing
                tunnel: w518 -> [w558]
                tunnel: [w556] -> w531
                stop <- w557 stop-if-true
                n196 = Not Equal?(x=w558, y=w556) -> (x != y?=w557:bool)
              }
              n197 = for {
                tunnel: w516 -> [w559] mode=indexing
                tunnel: w519 -> [w561]
                tunnel: [w559] -> w530
                stop <- w560 stop-if-true
                n198 = Not Equal?(x=w561, y=w559) -> (x != y?=w560:bool)
              }
              n199 = invoke class="Term" method="Connect Wire"(reference=w543, error in=w539, "Wire Source"=w542) -> (error out=w522:errorcluster)  [unwired: 4 in, 6 out]
              n200 = invoke class="Term" method="Connect Wire"(reference=w531, error in=w523, "Wire Source"=w530) -> (error out=w520:errorcluster)  [unwired: 4 in, 6 out]
              n201 = Merge Errors(w522, w520) -> (w521:errorcluster)
              n202 = invoke class="SubVI" method="Delete"(reference=w537, error in=w521) -> (error out=w538:errorcluster)  [unwired: 1 in, 2 out]
            }
          }
          n203 = Merge Errors(w334, w315, w298) -> (w289:errorcluster)
          n204 = Close Reference(reference=w292) -> ()  [unwired: 1 in, 1 out]
          n205 = Close Reference(reference=w301) -> ()  [unwired: 1 in, 1 out]
          n206 = Close Reference(reference=w296) -> ()  [unwired: 1 in, 1 out]
          n207 = Close Reference(reference=w299) -> ()  [unwired: 1 in, 1 out]
          n208 = flat-sequence {
            tunnel: [w444] -> w288
            tunnel: w289 -> [w444]
            tunnel: w322 -> [w443]
            frame #0 {
              n209 = Close Reference(reference=w443) -> ()  [unwired: 1 in, 1 out]
            }
          }
        }
      }
      n210 = invoke class="VI" method="BD.CleanUp"(reference=w53, error in=w91) -> (reference out=w90:refnum<vi>, error out=w88:errorcluster)  [unwired: 1 in, 1 out]
      n211 = property class="VI"(reference=w90, error in=w88, "Description"=w86) -> (reference out=w89:refnum<vi>, error out=w87:errorcluster)
      n212 = invoke class="VI" method="Save.Instrument"(reference=w89, error in=w87, "Path to saved file"=w61, "Save a Copy"=FALSE, "Without Diagram"=FALSE ("Save a Copy")) -> (reference out=w92:refnum<vi>, error out=w71:errorcluster)  [unwired: 1 in, 4 out]
      n213 = property class="LVClassLibrary"(reference=w75, error in=w71) -> (reference out=w69:refnum<vi>, error out=w77:errorcluster, "Children[]"=w76:refnum<vi>[])
      n214 = Strip Path(path=w61) -> (name=w64:string)  [unwired: 1 out]
      n215 = for {
        tunnel: w76 -> [w591] mode=indexing
        shift-right: [w585] -> w70
        shift-left: w77 -> [w590]
        tunnel: "Send Template.vi" -> [w589]
        shift-right: [w581] -> w63
        shift-left: FALSE -> [w580]
        tunnel: w64 -> [w584]
        n216 = property class="ProjectItem"(reference=w591, error in=w590) -> (reference out=w587:refnum<vi>, error out=w586:errorcluster, "Name"=w583:string)
        n217 = Equal?(x=w583, y=w584) -> (x = y?=w582:bool)
        n218 = Equal?(x=w583, y=w589) -> (x = y?=w588:bool)
        n219 = case shown="True" w588 {
          tunnel: w587 -> [_ w595]
          tunnel: w586 -> [w592 w594]
          tunnel: [w592 w593] -> w585
          frame False {
          }
          frame True {
            n220 = invoke class="ProjectItem" method="Delete"(reference=w595, error in=w594) -> (error out=w593:errorcluster)  [unwired: 1 in, 2 out]
          }
        }
        n221 = Select(t=TRUE, s=w582, f=w580) -> (s? t:f=w581:bool)
      }
      n222 = for {
        tunnel: w76 -> [w578] mode=indexing
        tunnel: w70 -> [_]
        n223 = Close Reference(reference=w578) -> ()  [unwired: 1 in, 1 out]
      }
      n224 = Strip Path(path=w61) -> (name=w66:string)  [unwired: 1 out]
      n225 = case shown="False" w63 {
        tunnel: "VI" ("Type") -> [w575 _]
        tunnel: w70 -> [w573 w576]
        tunnel: w69 -> [w572 w577]
        tunnel: [w571 w576] -> w68
        tunnel: [w570 w577] -> w67
        tunnel: w66 -> [w569 _]
        tunnel: w61 -> [w568 _]
        frame False {
          n226 = invoke class="LVClassLibrary" method="AddItem"(reference=w572, error in=w573, "Name"=w569, "Path"=w568, "Type"=w575) -> (reference out=w570:refnum<vi>, error out=w571:errorcluster, "AddItem"=w574:refnum<vi>)  [unwired: 1 in, 3 out]
          n227 = Close Reference(reference=w574) -> ()  [unwired: 1 in, 1 out]
        }
        frame True {
        }
      }
      n228 = Strip Path(path=w57) -> (name=w56:string)  [unwired: 1 out]
      n229 = invoke class="LVClassLibrary" method="Save"(reference=w67, error in=w68) -> (error out=w58:errorcluster)  [unwired: 2 in, 3 out]
      n230 = Equal?(x="Send Template.vi", y=w56) -> (x = y?=w54:bool)
      n231 = flat-sequence {
        tunnel: w92 -> [w111]
        tunnel: w57 -> [w110]
        tunnel: [w109] -> w59
        tunnel: w58 -> [w109]
        tunnel: w54 -> [w108]
        frame #0 {
          n232 = case shown="True" w108 {
            tunnel: w110 -> [_ w112]
            frame False {
            }
            frame True {
              n233 = Delete(path (use dialog)=w112) -> ()  [unwired: 4 in, 3 out]
            }
          }
          n234 = Close Reference(reference=w111) -> ()  [unwired: 1 in, 1 out]
        }
      }
    }
    frame Error {
    }
  }
  "error out" <- w47
